vi "GZip Compress.vi"(8 "error in (no error)":errorcluster, 11 "Uncompressed string":string="Hello World!") -> (0 "error out":errorcluster, 3 "GZip compressed string":string, 5 "Ratio":dbl)   [LabVIEW 2015, in "LSR Transmission.lvlib"]
doc: "Returns the GZip compressed value of the string input. Uses the Open G Zip Tools. Requires version 4.1.0-b2 or later for Linux RT support."
uses:
  LSR Transmission.lvlib
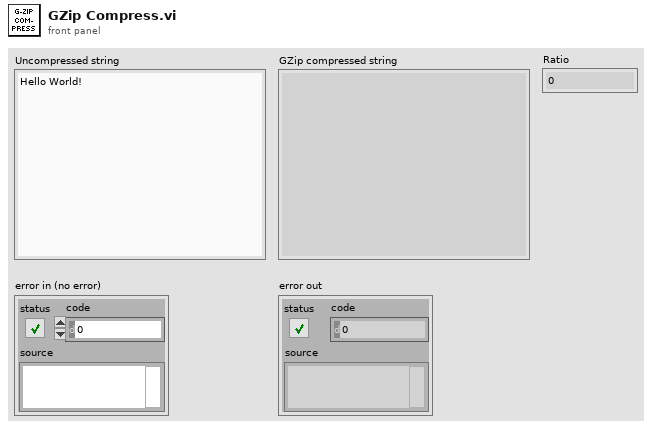
[diagram p1: front panel]
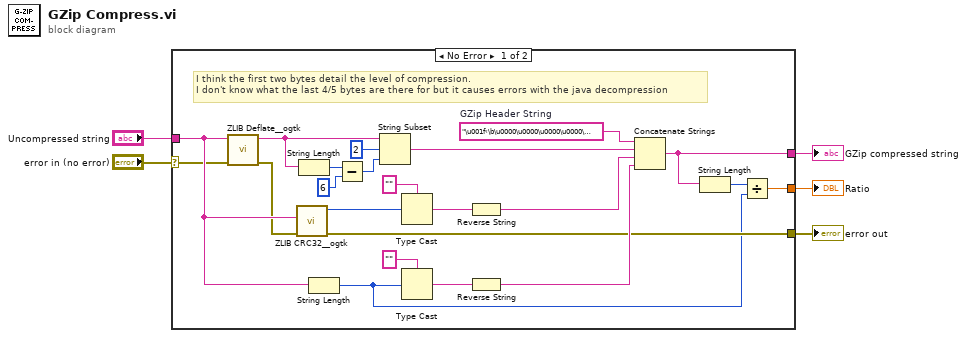
[diagram p0: block diagram]
diagram:
  n1 = case shown="No Error" "error in (no error)" {
    selector: "error in (no error)" -> [w10 w28]
    tunnel: "Uncompressed string" -> [w22 _]
    tunnel: [w15 w28] -> w4
    tunnel: [w14 _] -> w3
    tunnel: [w11 _] -> w2
    frame No Error {
      w17 = "\u001f‹\b\u0000\u0000\u0000\u0000\u0000\u0004\u0000"  # GZip Header String
      # "I think the first two bytes detail the level of compression.\nI don't know what the last 4/5 bytes are there for but it causes errors with the java decompression"
      n2 = call <userlib>:"ZLIB Deflate__ogtk.vi"("error in (no error)"=w10, "input"=w22) -> ("error out"=w16:errorcluster, "deflated output"=w9:string)  [unwired: 3 in, 1 out]
      n3 = call <userlib>:"ZLIB CRC32__ogtk.vi"("error in (no error)"=w16, "buffer"=w22) -> ("error out"=w15:errorcluster, "new crc32"=w20:u32)  [unwired: 4 in]
      n4 = String Length(string=w9) -> (length=w8:i32)
      n5 = String Length(string=w22) -> (length=w12:i32)
      n6 = Subtract(x=w8, y=6) -> (x-y=w7:i32)
      n7 = String Subset(string=w9, offset (0)=2, length (rest)=w7) -> (substring=w19:string)
      n8 = Type Cast(type="", x=w20) -> (*(type *) &x=w24:string)
      n9 = Type Cast(type="", x=w12) -> (*(type *) &x=w25:string)
      n10 = Reverse String(1:w24) -> (0:w26:string)
      n11 = Reverse String(1:w25) -> (0:w27:string)
      n12 = Concatenate Strings(w17, w19, w26, w27) -> (w14:string)
      n13 = String Length(string=w14) -> (length=w13:i32)
      n14 = Divide(x=w13, y=w12) -> (x/y=w11:dbl)
    }
    frame Error {
    }
  }
  "GZip compressed string" <- w3
  "error out" <- w4
  "Ratio" <- w2
